vi "A34401Configure Multipoint.vi"(5 "Sample Source (0:Trigger Delay)":u16(ring) items=["Trigger Delay", "Sample Interval"], 6 "Sample Interval (0.1 seconds)":dbl=0.1, 7 "Pretrigger Samples (0)":i32, 8 "error in (no error)":errorcluster, 9 "Sample Count (1)":i32=1 format="%#.6g", 10 "Trigger Count (1)":i32=1 format="%#.6g", 11 "VISA resource name":refnum<visa-resource-name>) -> (0 "error out":errorcluster, 3 "VISA resource name out":refnum<visa-resource-name>)   [LabVIEW 2019, in "A34401Agilent 34401.lvlib"]
doc: "Configures trigger count, pretrigger count, sample interval, and sample count so you can take multi-point measurements.\n\n<B>Note:</B>\n- This VI will only be used with the low level Data VIs, as the high level VIs already contain this functionality. \n- Due to instrument limitations, the 34410 does not support <B>Pretrigger Samples</B> and the 34401 model does not support the setting of <B>Pretrigger Samples</B> or <B>Sample Interval</B>."
uses:
  A34401Agilent 34401.lvlib
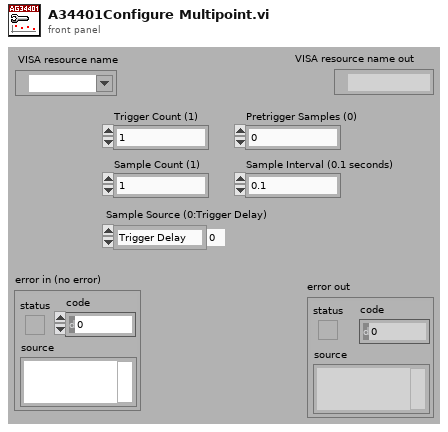
[diagram p1: front panel]
types:
  T1 = typedef "A34401Agilent 34401.lvlib/A34401Extended User Data.ctl" = cluster{"Trigger Source":u16, "Math Storage":u16, "Agilent Model":i32}
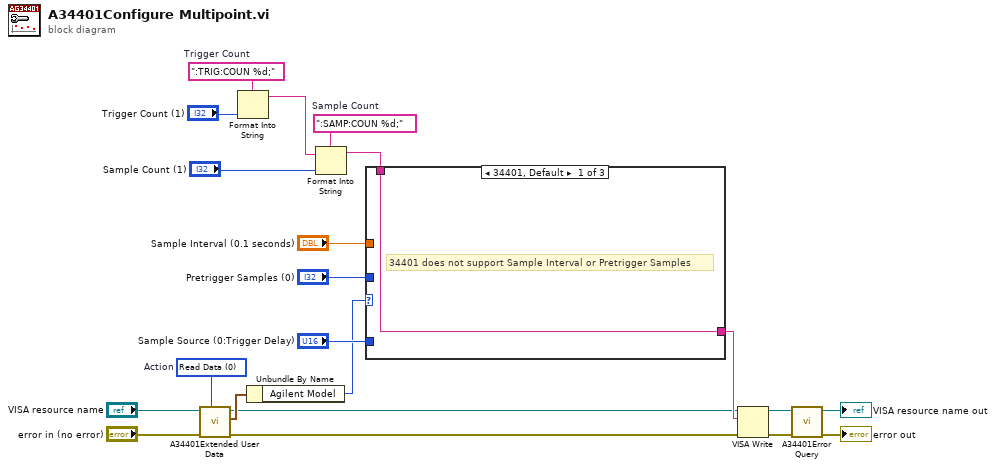
[diagram p0: block diagram]
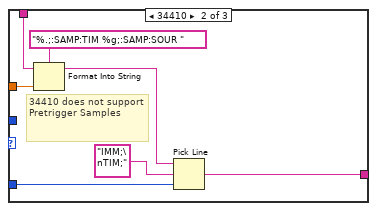
[diagram p2: hidden frame]
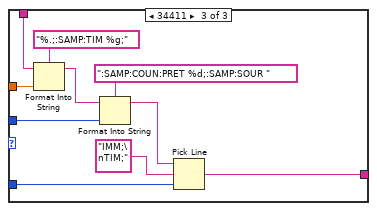
[diagram p3: hidden frame]
diagram:
  w7 = u16 0 items=["Read Data", "Write Data", "Dispose of Data"]  # Action
  w15 = ":SAMP:COUN %d;"  # Sample Count
  w16 = ":TRIG:COUN %d;"  # Trigger Count
  n1 = call "A34401Extended User Data.vi"("Action (0: Read Data)"=w7, "Error In (no error)"="error in (no error)", "VISA resource name in"="VISA resource name") -> ("Error Out"=w3:errorcluster, "User Data Out"=w6:T1, "VISA resource name out"=w2:refnum<visa-resource-name>)  [unwired: 6 in]
  n2 = Format Into String(format string=w16, "Trigger Count (1)") -> (resulting string=w13:string)  [unwired: 2 in, 1 out]
  n3 = Unbundle By Name(w6) -> ("Agilent Model"=w1:i32)
  n4 = Format Into String(format string=w15, initial string=w13, "Sample Count (1)") -> (resulting string=w12:string)  [unwired: 1 in, 1 out]
  n5 = case shown="34401, Default" w1 {
    tunnel: w12 -> [w22 w27 w38]
    tunnel: [w22 w24 w33] -> w11
    tunnel: "Sample Interval (0.1 seconds)" -> [_ w28 w39]
    tunnel: "Pretrigger Samples (0)" -> [_ _ w34]
    tunnel: "Sample Source (0:Trigger Delay)" -> [_ w25 w31]
    frame 34401, Default {
      # "34401 does not support Sample Interval or Pretrigger Samples"
    }
    frame 34410 {
      # "34410 does not support Pretrigger Samples"
      n6 = Format Into String(format string="%.;:SAMP:TIM %g;:SAMP:SOUR ", initial string=w27, w28) -> (resulting string=w23:string)  [unwired: 1 in, 1 out]
      n7 = Pick Line(string ("")=w23, multi-line string="IMM;\nTIM;", line index=w25) -> (output string=w24:string)
    }
    frame 34411 {
      n8 = Format Into String(format string="%.;:SAMP:TIM %g;", initial string=w38, w39) -> (resulting string=w36:string)  [unwired: 1 in, 1 out]
      n9 = Format Into String(format string=":SAMP:COUN:PRET %d;:SAMP:SOUR ", initial string=w36, w34) -> (resulting string=w32:string)  [unwired: 1 in, 1 out]
      n10 = Pick Line(string ("")=w32, multi-line string="IMM;\nTIM;", line index=w31) -> (output string=w33:string)
    }
  }
  n11 = VISA Write(VISA resource name=w2, write buffer=w11, error in (no error)=w3) -> (VISA resource name out=w19:refnum<visa-resource-name>, error out=w18:errorcluster)  [unwired: 1 out]
  n12 = call "A34401Error Query.vi"("error in (no error)"=w18, "VISA resource name"=w19) -> ("error out"=→"error out":errorcluster, "VISA resource name out"=→"VISA resource name out":refnum<visa-resource-name>)  [unwired: 6 in, 2 out]
